vi "Speed Turn Math.vi"(0 "Throttle":dbl, 1 "Lower Turn Speed":dbl, 3 "Upper Turn Speed":dbl, 5 "Turn":dbl, 9 "Maximum Linear Speed":dbl, 11 "Scale Intertia":dbl=0.02) -> (4 "Left Wheel Velocity":dbl, 8 "Right Wheel Velocity":dbl)   [LabVIEW 2017]
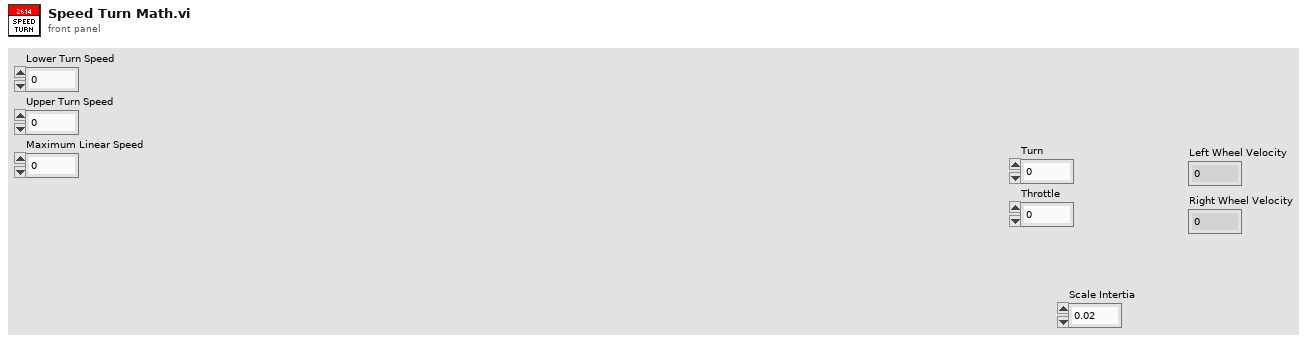
[diagram p1: front panel]
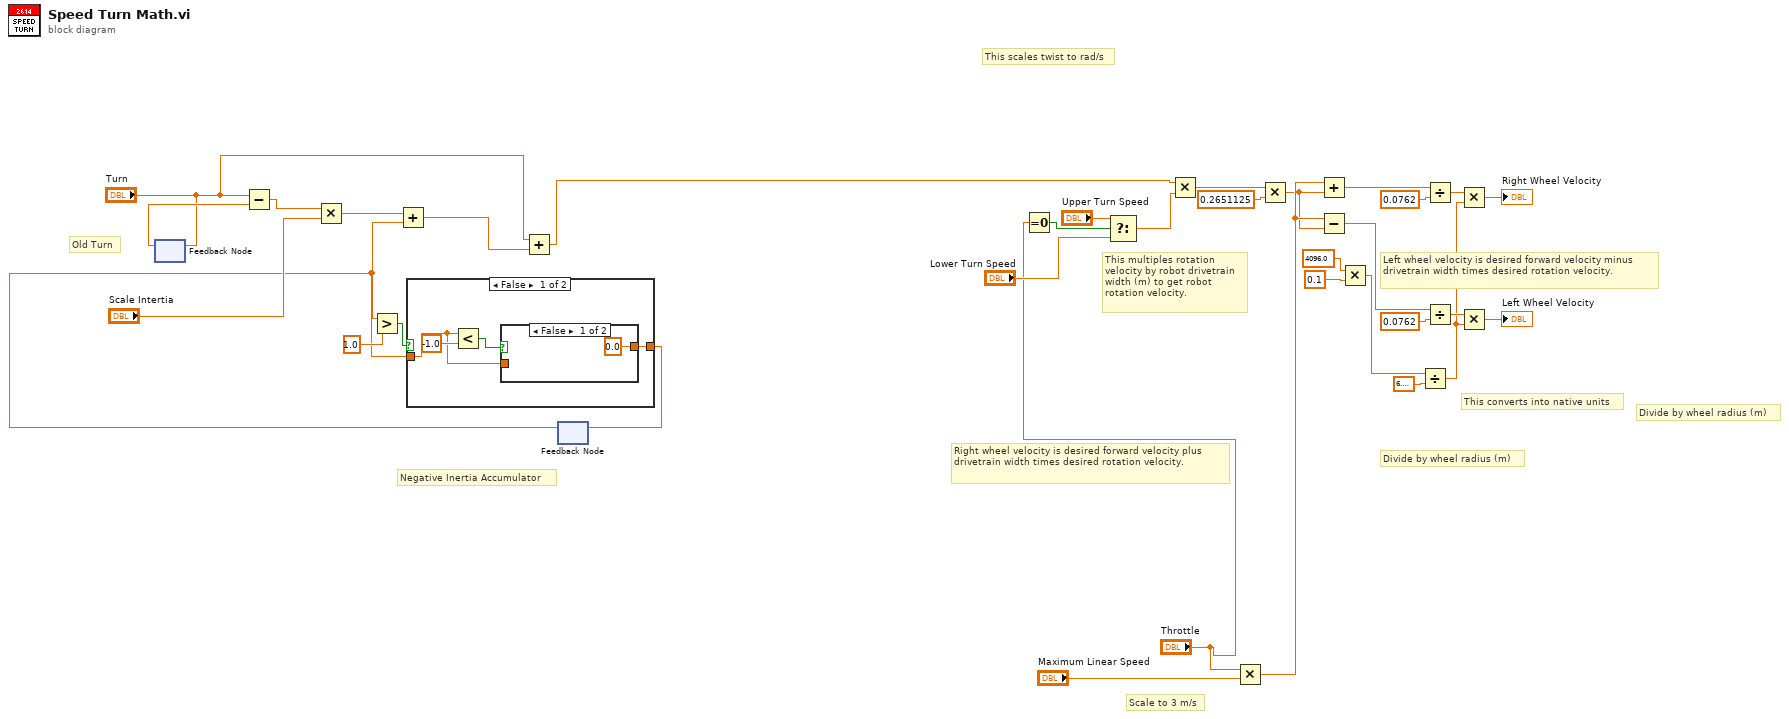
[diagram p0: block diagram]
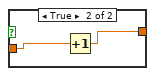
[diagram p2: hidden frame]
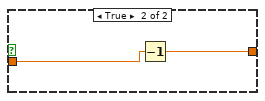
[diagram p3: hidden frame]
diagram:
  # "Old Turn"
  # "Negative Inertia Accumulator"
  # "This converts into native units"
  # "Divide by wheel radius (m)"
  # "Divide by wheel radius (m)"
  # "Right wheel velocity is desired forward velocity plus drivetrain width times desired rotation velocity."
  # "This multiples rotation velocity by robot drivetrain width (m) to get robot rotation velocity."
  # "Left wheel velocity is desired forward velocity minus  drivetrain width times desired rotation velocity."
  # "This scales twist to rad/s"
  # "Scale to 3 m/s"
  n1 = feedback-in #1("Turn") -> ()
  n2 = feedback #1() -> (w3:dbl)  [unwired: 1 in]
  n3 = Subtract(x="Turn", y=w3) -> (x-y=w17:dbl)
  n4 = Multiply(x=w17, y="Scale Intertia") -> (x*y=w15:dbl)
  n5 = feedback #2() -> (w4:dbl)  [unwired: 1 in]
  n6 = Greater?(x=w4, y=1.0) -> (0:w11:bool)
  n7 = Add(x=w15, y=w4) -> (x+y=w14:dbl)
  n8 = case shown="False" w11 {
    tunnel: w4 -> [w36 w43]
    tunnel: [w35 w42] -> w5
    frame False {
      n9 = Less?(x=w36, y=-1.0) -> (x < y?=w37:bool)
      n10 = case shown="False" w37 {
        tunnel: w36 -> [_ w41]
        tunnel: [0.0 w40] -> w35
        frame False {
        }
        frame True {
          n11 = Increment(x=w41) -> (x+1=w40:dbl)
        }
      }
    }
    frame True {
      n12 = Decrement(x=w43) -> (x-1=w42:dbl)
    }
  }
  n13 = Add(x="Turn", y=w14) -> (x+y=w13:dbl)
  n14 = feedback-in #2(w5) -> ()
  n15 = Equal To 0?(x="Throttle") -> (x = 0?=w9:bool)
  n16 = Select(t="Upper Turn Speed", s=w9, f="Lower Turn Speed") -> (s? t:f=w10:dbl)
  n17 = Multiply(x=w13, y=w10) -> (x*y=w34:dbl)
  n18 = Multiply(x="Throttle", y="Maximum Linear Speed") -> (x*y=w32:dbl)
  n19 = Multiply(x=w34, y=0.2651125) -> (x*y=w31:dbl)
  n20 = Add(x=w32, y=w31) -> (x+y=w30:dbl)
  n21 = Subtract(x=w32, y=w31) -> (x-y=w29:dbl)
  n22 = Multiply(x=4096.0, y=0.1) -> (x*y=w20:dbl)
  n23 = Divide(x=w20, y=6.283185307179586) -> (x/y=w18:dbl)
  n24 = Divide(x=w30, y=0.0762) -> (x/y=w23:dbl)
  n25 = Divide(x=w29, y=0.0762) -> (x/y=w24:dbl)
  n26 = Multiply(x=w23, y=w18) -> (x*y=→"Right Wheel Velocity":dbl)
  n27 = Multiply(x=w24, y=w18) -> (x*y=→"Left Wheel Velocity":dbl)
